vi "SF2 Video Processing Target Detection.vi"(7 "Update":bool, 10 "Vision Angle (in)":dbl format="%#_13g", 11 "Timestamp (in)":u32) -> (1 "New Data Avaliable":bool, 2 "Vision Angle (out)":dbl, 3 "Timestamp (out)":u32)   [LabVIEW 2016]
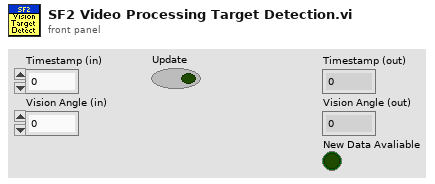
[diagram p1: front panel]
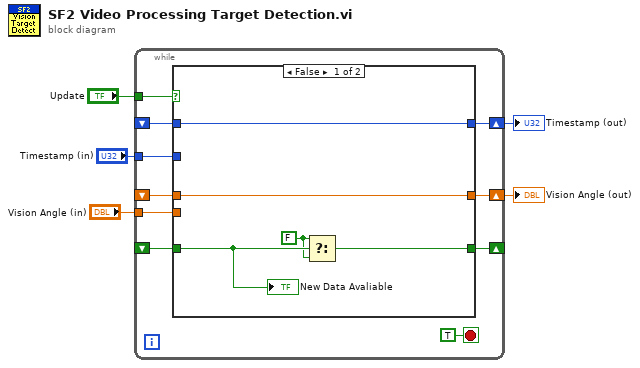
[diagram p0: block diagram]
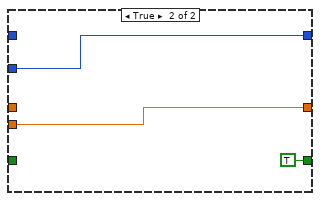
[diagram p2: hidden frame]
diagram:
  n1 = while {
    tunnel: "Update" -> [w15]
    shift-right: [w13] -> w4
    shift-left: _ -> [w12]
    tunnel: "Timestamp (in)" -> [w14]
    shift-right: [w10] -> w2
    shift-left: _ -> [w11]
    tunnel: "Vision Angle (in)" -> [w9]
    shift-right: [w7] -> _
    shift-left: _ -> [w8]
    stop <- TRUE stop-if-true
    n2 = case shown="False" w15 {
      tunnel: w14 -> [_ w23]
      tunnel: [w20 w23] -> w13
      tunnel: w12 -> [w20 _]
      tunnel: [w19 w22] -> w10
      tunnel: w11 -> [w19 _]
      tunnel: w9 -> [_ w22]
      tunnel: w8 -> [w17 _]
      tunnel: [w18 TRUE] -> w7
      frame False {
        w16 = FALSE
        n3 = Select(t=w16, s=w17, f=w16) -> (s? t:f=w18:bool)
        "New Data Avaliable" <- w17
      }
      frame True {
      }
    }
  }
  "Timestamp (out)" <- w4
  "Vision Angle (out)" <- w2
